vi "Read Triggered Voltage Level.vi"(0 "VISA resource name":refnum<visa-resource-name>, 11 "error in (no error)":errorcluster) -> (4 "VISA resource name out":refnum<visa-resource-name>, 6 "Measurement":string, 15 "error out":errorcluster)   [LabVIEW 2018, in "Keithley KE22xx Series.lvlib"]
doc: "Read the response from the instrument for the set value of Triggered Voltage level."
uses:
  Keithley KE22xx Series.lvlib
panel:
  # "© 2012 Keithley Instruments, Inc. ALL RIGHTS RESERVED"
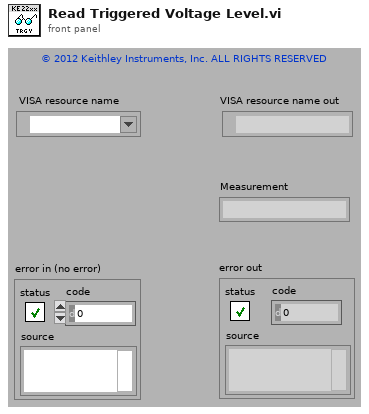
[diagram p1: front panel]
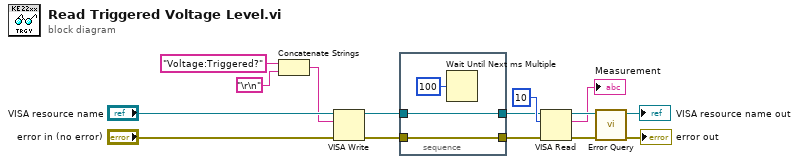
[diagram p0: block diagram]
diagram:
  n1 = Concatenate Strings("Voltage:Triggered?", "\r\n") -> (w3:string)
  n2 = VISA Write(VISA resource name="VISA resource name", write buffer=w3, error in (no error)="error in (no error)") -> (VISA resource name out=w5:refnum<visa-resource-name>, error out=w4:errorcluster)  [unwired: 1 out]
  n3 = stacked-sequence {
    tunnel: [w18] -> w10
    tunnel: w5 -> [w18]
    tunnel: w4 -> [w17]
    tunnel: [w17] -> w9
    frame #0 {
      n4 = Wait Until Next ms Multiple(millisecond multiple=u32 100 ("Programmable Delay in ms")) -> ()  [unwired: 1 out]
    }
  }
  n5 = VISA Read(VISA resource name=w10, byte count=u32 10, error in (no error)=w9) -> (VISA resource name out=w13:refnum<visa-resource-name>, read buffer=→"Measurement":string, error out=w12:errorcluster)  [unwired: 1 out]
  n6 = call "Error Query.vi"("error in (no error)"=w12, "VISA resource name"=w13) -> ("error out"=→"error out":errorcluster, "VISA resource name out"=→"VISA resource name out":refnum<visa-resource-name>)  [unwired: 6 in, 2 out]
